vi "AddFragment.vi"(8 "error in (no error)":errorcluster, 10 "Fragment":string, 11 "MsgPackSerializer in":refnum<class "MsgPackSerializer.lvclass">) -> (0 "error out":errorcluster, 3 "MsgPackSerializer out":refnum<class "MsgPackSerializer.lvclass">)   [LabVIEW 2015, in "MsgPackSerializer.lvclass"]
uses:
  MsgPackSerializer.lvclass
  Fragment.ctl
  MsgPackSerializer.lvclass/MsgPackSerializer.ctl
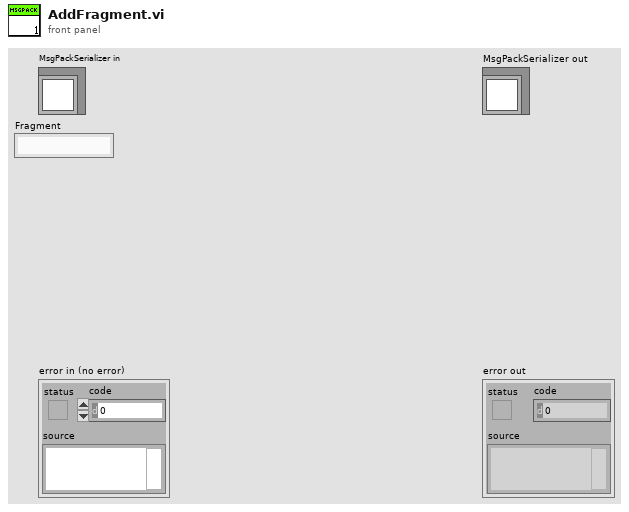
[diagram p1: front panel]
types:
  T1 = typedef "MsgPackSerializer.lvclass/Fragment.ctl" = cluster{"DVR":refnum<data-value>, "Length":i64}
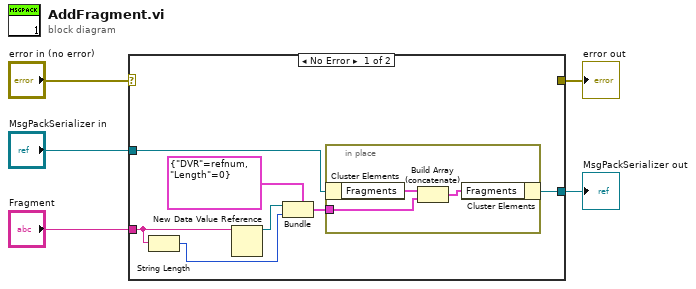
[diagram p0: block diagram]
diagram:
  n1 = case shown="No Error" "error in (no error)" {
    selector: "error in (no error)" -> [_ w17]
    tunnel: [_ w17] -> w4
    tunnel: [w11 w16] -> w2
    tunnel: "MsgPackSerializer in" -> [w12 w16]
    tunnel: "Fragment" -> [w7 _]
    frame No Error {
      n2 = String Length(string=w7) -> (length=w9:i32)
      n3 = New Data Value Reference(data value=w7) -> (data value reference=w8:refnum<data-value>)  [unwired: 1 in, 1 out]
      n4 = Bundle(cluster=T1 {"DVR"=refnum, "Length"=0} ("Fragment"), "DVR"=w8, "Length"=w9) -> (w6:T1)
      n5 = in-place {
        in-place-border: w6 -> [w14]
        n6 = in-place-cluster #1(w12) -> ("Fragments"=w15:T1[])
        n7 = Build Array (concatenate)(w15, w14) -> (w13:T1[])
        n8 = in-place-cluster #1("Fragments"=w13) -> (w11:refnum<class "MsgPackSerializer.lvclass">)
      }
    }
    frame Error {
    }
  }
  "error out" <- w4
  "MsgPackSerializer out" <- w2
